vi "Set Measurement.vi"(8 "error in (no error)":errorcluster, 9 "conversion (0 : off)":u16(ring) items=["off", "Z: Ref1", "Z: Trans", "Y: Ref1", "Y: trans", "1/S"], 10 "measurement (0 : S11)":u16(ring) items=["Ref1 : Forward S11 (A/R)", "Trans: Forward S21 (B/R)", "Trans: Reverse S12 (A/R)", "Ref1: Reverse S22 (B/R)", "Analog In, AUX input", "A/R", "B/R", "A/B", "A", "B", "R"], 11 "VISA resource name":refnum<visa-resource-name>) -> (0 "error out":errorcluster, 3 "VISA resource name out":refnum<visa-resource-name>)   [LabVIEW 2018, in "Agilent 87XX Series.lvlib"]
doc: "This VI for the HP8753B Network Analyzer sets the measurement."
uses:
  Agilent 87XX Series.lvlib
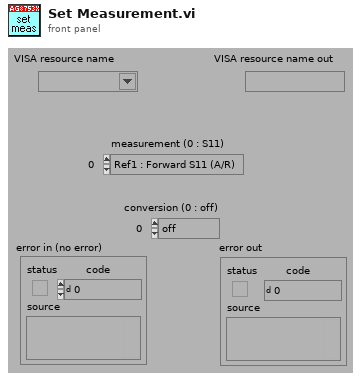
[diagram p1: front panel]
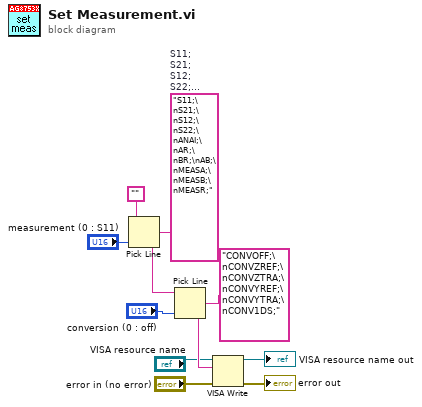
[diagram p0: block diagram]
diagram:
  w5 = "S11;\nS21;\nS12;\nS22;\nANAI;\nAR;\nBR;\nAB;\nMEASA;\nMEASB;\nMEASR;"  # S11; S21; S12; S22; ANAI; AR; BR; AB; MEASA; MEASB; MEASR;
  n1 = Pick Line(string ("")="", multi-line string=w5, line index="measurement (0 : S11)") -> (output string=w4:string)
  n2 = Pick Line(string ("")=w4, multi-line string="CONVOFF;\nCONVZREF;\nCONVZTRA;\nCONVYREF;\nCONVYTRA;\nCONV1DS;", line index="conversion (0 : off)") -> (output string=w9:string)
  n3 = VISA Write(VISA resource name="VISA resource name", write buffer=w9, error in (no error)="error in (no error)") -> (VISA resource name out=→"VISA resource name out":refnum<visa-resource-name>, error out=→"error out":errorcluster)  [unwired: 1 out]
